vi "MovCor-Update some FGV values when ref selected.vi"(6 "Threshold":i16[](array[numeric]), 9 "Reference Rectangles":i16[][](array[numeric]), 10 "AOL Z":dbl, 11 "Reference image":T1) -> (0 "error out":errorcluster)   [LabVIEW 2020]
uses:
  <vilib>/vision/Image Controls.llb/IMAQ Image.ctl
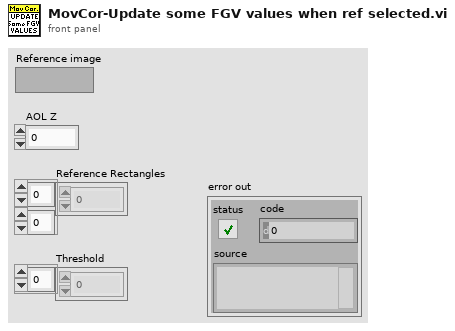
[diagram p1: front panel]
types:
  T1 = typedef "IMAQ Image.ctl" = refnum<image>
  T2 = typedef "Ref DAQ Param.ctl" = cluster{"Full Frame Size":u16, "Ref Field of View":sgl, "Ref Zoom":i8, "Ref_dwellTime":sgl, "Ref X-pixels-per-line(Npxr)":i16, "Ref Y-lines-per-image(Npyr)":i16, "Ref Z-lines-per-image":i16, "Ignore Z lines":i16, "Ref Scan Cycles":i32, "Ref threshold XY":u16, "Ref threshold Z":u16, "Ref average XY":u16, "Ref Average  Z":u16, "Proportional_scale":fxp<+,16,2>, "Integral_scale":fxp<+/-,16,12>, "Proportional_scale Z":fxp<+,16,2>, "Integral_scale Z":fxp<+/-,16,12>, "Diff_threshold":fxp<+,16,2>, "Diff_threshold _z":fxp<+,16,2>, "Sliding Average":bool, "Ref count reset enabled":bool}
  T3 = typedef "Reference_Globals.ctl" = cluster{"Refrence data path":path, "Reference Rectangle":i16[][], "AOL Z":dbl, "No of pixels in a miniscan ":i32[], "Threshold":i16[], "No of miniscans":i32[], "Full Frame Size":u16, "Reference Image":T1, "dwelltime":dbl, "Zoom":dbl, "Field of View":dbl, "Z Step":i8, "Z pixels":i32, "Z Lines":u8, "Z Ignore":u8, "Laser":u8}
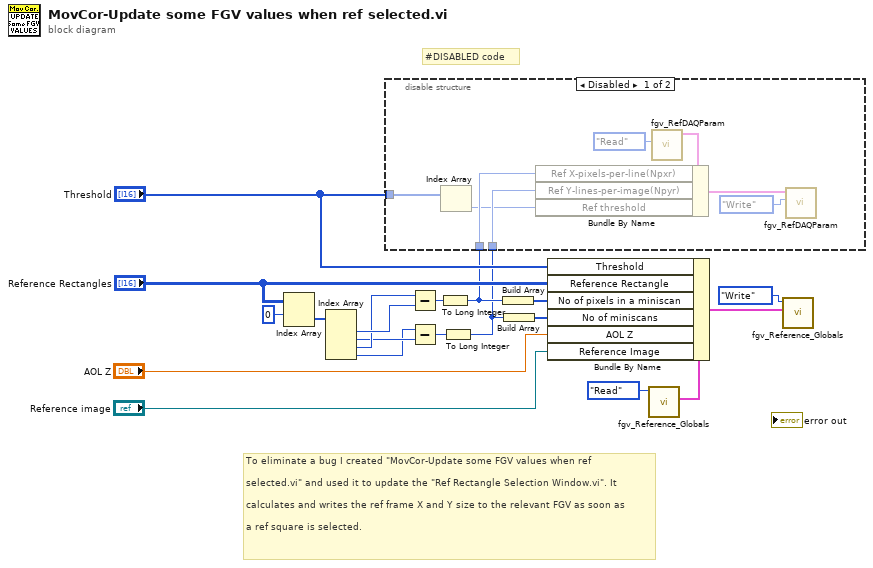
[diagram p0: block diagram]
diagram:
  # "#DISABLED code"
  # "To eliminate a bug I created \"MovCor-Update some FGV values when ref \n\nselected.vi\" and used it to update the \"Ref Rectangle Selection Window.vi\". It \n\ncalculates and writes the ref frame X and Y size to the relevant FGV as soon as \n\na ref square is selected."
  n1 = Index Array(array="Reference Rectangles", index (row)=0) -> (element=w1:i16[])  [unwired: 1 in]
  n2 = Index Array(array=w1) -> (element #1=w7:i16, element #2=w3:i16, element #3=w5:i16, element #4=w2:i16)  [unwired: 4 in]
  n3 = Subtract(x=w5, y=w7) -> (x-y=w6:i16)
  n4 = Subtract(x=w2, y=w3) -> (x-y=w4:i16)
  n5 = To Long Integer(number=w6) -> (32bit integer=w15:i32)
  n6 = To Long Integer(number=w4) -> (32bit integer=w14:i32)
  n7 = disable-structure shown="Disabled" {
    disable-tunnel: "Threshold" -> [w28 _]
    disable-tunnel: w15 -> [w26 _]
    disable-tunnel: w14 -> [w25 _]
    frame Disabled {
      n8 = Index Array(array=w28) -> (element=w24:i16)  [unwired: 1 in]
      n9 = call "fgv_RefDAQParam.vi"("Function"=enum16{"Initialize", "Write", "Read"}."Read" ("Status")) -> ("RefDAQParam"=w23:T2)  [unwired: 9 in, 1 out]
      n10 = Bundle By Name(cluster=w23, "Ref X-pixels-per-line(Npxr)"=w26, "Ref Y-lines-per-image(Npyr)"=w25, "Ref threshold"=w24) -> (w27:T2)
      n11 = call "fgv_RefDAQParam.vi"("Function"=enum16{"Initialize", "Write", "Read"}."Write" ("Status"), "RefDAQParam in"=w27) -> ()  [unwired: 8 in, 2 out]
    }
    frame Enabled {
    }
  }
  n12 = Build Array(w15) -> (w11:i32[])
  n13 = Build Array(w14) -> (w12:i32[])
  n14 = call "fgv_Reference_Globals.vi"("Function"=enum16{"Intialize", "Write", "Read", "Clear"}."Read") -> ("Reference Data"=w16:T3)  [unwired: 9 in, 1 out]
  n15 = Bundle By Name(cluster=w16, "Threshold"="Threshold", "Reference Rectangle"="Reference Rectangles", "No of pixels in a miniscan"=w11, "No of miniscans"=w12, "AOL Z"="AOL Z", "Reference Image"="Reference image") -> (w10:T3)
  n16 = call "fgv_Reference_Globals.vi"("Reference Data"=w10, "Function"=enum16{"Intialize", "Write", "Read", "Clear"}."Write") -> ()  [unwired: 8 in, 2 out]
